vi "Recipe Builder.vi"() -> ()   [LabVIEW 2017, in "Recipes.lvclass"]
uses:
  Recipes.lvclass
  Type Defs/Recipes Queue Element.ctl
  Type Defs/Recipes State.ctl
panel:
  in  "Create New":bool
  in  "Recipe Mode":enum32{"Saturation", "Expansion", "Both"}(radio)
  in  "Other Settings":cluster{"Name":string, "Value":string}[](array[cluster])
  in  "Edit Recipe":bool
  in  "Load Recipe":bool
  in  "Apply Changes":bool
  in  "Saturation Time":string
  in  "Expansion Time":string
  in  "Recipes":i32(listbox)
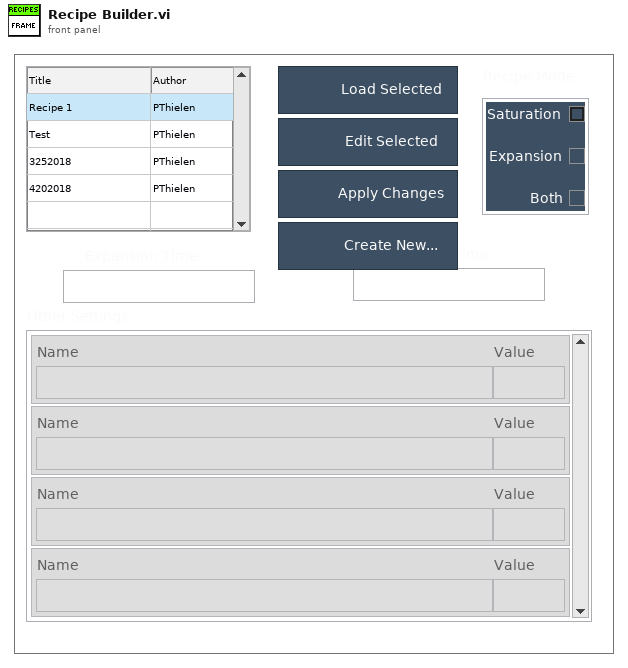
[diagram p1: front panel]
types:
  T1 = typedef "Recipes.lvclass/Recipes Queue Element.ctl" = cluster{"State":T2, "Variant":variant}
  T2 = typedef "Recipes.lvclass/Recipes State.ctl" = enum16{"Init", "Go", "Stop", "Idle", "Error", "Shutdown"}
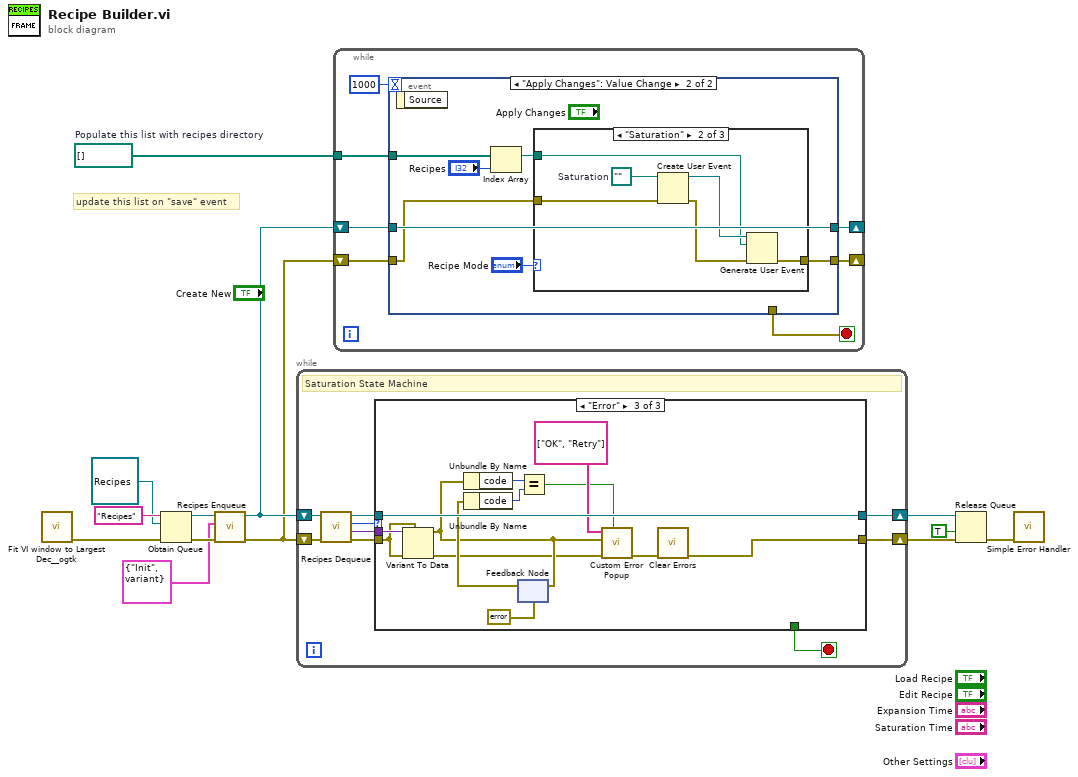
[diagram p0: block diagram]
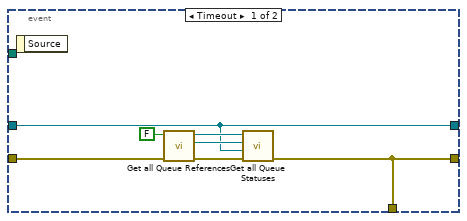
[diagram p2: hidden frame]
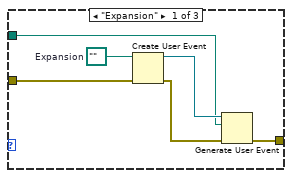
[diagram p3: hidden frame]
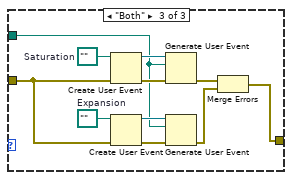
[diagram p4: hidden frame]
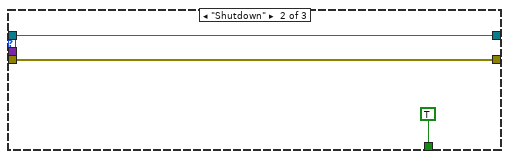
[diagram p6: hidden frame]
diagram:
  w1 = path[] []  # Populate this list with recipes directory
  # "update this list on \"save\" event"
  n1 = call "Fit VI window to Largest Dec__ogtk.vi"() -> ("error out"=w8:errorcluster)  [unwired: 6 in, 1 out]
  n2 = Obtain Queue(name (unnamed)="Recipes", element data type=refnum<class "Recipes.lvclass"> refnum ("Expansion.lvclass"), error in (no error)=w8) -> (queue out=w10:refnum<queue>, error out=w9:errorcluster)  [unwired: 2 in, 1 out]
  n3 = call "Recipes Enqueue.vi"("error in (no error)"=w9, "Expansion Queue Element"=T1 {"State"=enum."Init", "Variant"=variant}, "Queue in"=w10) -> ("error out"=w3:errorcluster, "Queue out"=w4:refnum<queue>)  [unwired: 7 in]
  n4 = while {
    shift-right: [w18] -> w12
    shift-left: w3 -> [w21]
    shift-right: [w16] -> w13
    shift-left: w4 -> [w22]
    stop <- w17 stop-if-true
    # "Saturation State Machine"
    n5 = call "Recipes Dequeue.vi"("error in (no error)"=w21, "Queue in"=w22) -> ("error out"=w19:errorcluster, "Data"=w14:variant, "State"=w15:T2, "Queue out"=w20:refnum<queue>)  [unwired: 6 in]
    n6 = case shown="\"Error\"" w15 {
      tunnel: w20 -> [w23 w26 w40]
      tunnel: w19 -> [w24 w27 w30]
      tunnel: [w24 w27 w37] -> w18
      tunnel: [_ TRUE _] -> w17
      tunnel: [w23 w26 w40] -> w16
      tunnel: w14 -> [_ _ w31]
      frame "Idle", Default {
      }
      frame "Shutdown" {
      }
      frame "Error" {
        n7 = Variant To Data(error in=w30, type=w30, Variant=w31) -> (data=w29:errorcluster, error out=w28:errorcluster)
        n8 = Unbundle By Name(w29) -> ("code"=w35:i32)
        n9 = feedback-in #1(w29) -> ()
        n10 = feedback #1(errorcluster {"status"=FALSE, "code"=0, "source"=""} ("error out")) -> (w36:errorcluster)
        n11 = Unbundle By Name(w36) -> ("code"=w34:i32)
        n12 = Equal?(x=w35, y=w34) -> (x = y?=w33:bool)
        n13 = call "Custom Error Popup.vi"("Repeated error?"=w33, "VI Error in"=w28, "Error to display"=w29, "Button Labels"=string[] ["OK", "Retry"]) -> ("error out"=w39:errorcluster)  [unwired: 6 in, 1 out]
        n14 = call <vilib>:"Clear Errors.vi"("error in (no error)"=w39) -> ("error out"=w37:errorcluster)  [unwired: 5 in, 1 out]
      }
    }
  }
  n15 = while {
    shift-right: [w44] -> _
    shift-left: w3 -> [w46]
    shift-right: [w43] -> _
    shift-left: w4 -> [w47]
    tunnel: w1 -> [w41]
    stop <- w45 stop-if-true
    n16 = event shown="[1] \"Apply Changes\": Value Change" {
      selector: _ -> [_ _]
      dyn-events: _ -> [_ _]
      timeout: 1000 -> [_ _]
      tunnel: w47 -> [w49 w61]
      tunnel: w46 -> [w53 w59]
      tunnel: [w52 _] -> w45
      tunnel: [w52 w60] -> w44
      tunnel: [w49 w61] -> w43
      tunnel: w41 -> [_ w57]
      event Timeout {
        n17 = event-data() -> ()  [unwired: 1 in, 1 out]
        n18 = call "Get all Queue References.vi"("error in (no error)"=w53, "create if not found? (F)"=FALSE ("create if not found? (T)")) -> ("error out"=w50:errorcluster, "Saturation Queue"=w54:refnum<queue>, "Expansion Queue"=w51:refnum<queue>)  [unwired: 6 in, 1 out]
        n19 = call "Get all Queue Statuses.vi"("error in (no error)"=w50, "Recipes Queue"=w49, "Saturation Queue"=w54, "Queue in"=w51) -> ("error out"=w52:errorcluster)  [unwired: 7 in]
      }
      event "Apply Changes": Value Change {
        n20 = event-data() -> ()  [unwired: 1 in, 1 out]
        n21 = Index Array(array=w57, index="Recipes") -> (element=w56:path)
        n22 = case shown="\"Saturation\"" "Recipe Mode" {
          tunnel: [w67 w73 w75] -> w60
          tunnel: w59 -> [w63 w69 w77]
          tunnel: w56 -> [w62 w68 w76]
          frame "Expansion" {
            w66 = path ""  # Expansion
            n23 = Create User Event(user event datatype=w66, error in=w63) -> (user event=w65:refnum<user-event>, error out=w64:errorcluster)
            n24 = Generate User Event(user event=w65, event data cluster=w62, error in=w64) -> (error out=w67:errorcluster)  [unwired: 1 in, 1 out]
          }
          frame "Saturation" {
            w72 = path ""  # Saturation
            n25 = Create User Event(user event datatype=w72, error in=w69) -> (user event=w71:refnum<user-event>, error out=w70:errorcluster)
            n26 = Generate User Event(user event=w71, event data cluster=w68, error in=w70) -> (error out=w73:errorcluster)  [unwired: 1 in, 1 out]
          }
          frame "Both" {
            w78 = path ""  # Expansion
            w83 = path ""  # Saturation
            n27 = Create User Event(user event datatype=w83, error in=w77) -> (user event=w82:refnum<user-event>, error out=w81:errorcluster)
            n28 = Create User Event(user event datatype=w78, error in=w77) -> (user event=w79:refnum<user-event>, error out=w80:errorcluster)
            n29 = Generate User Event(user event=w82, event data cluster=w76, error in=w81) -> (error out=w84:errorcluster)  [unwired: 1 in, 1 out]
            n30 = Generate User Event(user event=w79, event data cluster=w76, error in=w80) -> (error out=w74:errorcluster)  [unwired: 1 in, 1 out]
            n31 = Merge Errors(w84, w74) -> (w75:errorcluster)
          }
        }
      }
    }
  }
  n32 = Release Queue(queue=w13, force destroy? (F)=TRUE, error in (no error)=w12) -> (error out=w5:errorcluster)  [unwired: 2 out]
  n33 = call <vilib>:"Simple Error Handler.vi"("error in (no error)"=w5) -> ()  [unwired: 4 in, 5 out]
